vi "Write TDMS.vi"(8 "error in (no error)":errorcluster, 9 "Timed out? (False)":bool, 10 "Distance (m)":dbl, 11 "Parallax PING))) in":refnum<class "Parallax PING))).lvclass">) -> (0 "error out":errorcluster, 3 "Parallax PING))) out":refnum<class "Parallax PING))).lvclass">)   [LabVIEW 2013, in "Parallax PING))).lvclass"]
doc: "Writes data to the tdms file. Call Open TDMS VI before running this VI."
uses:
  Parallax PING))).lvclass
  Parallax PING))).lvclass/Parallax PING))).ctl
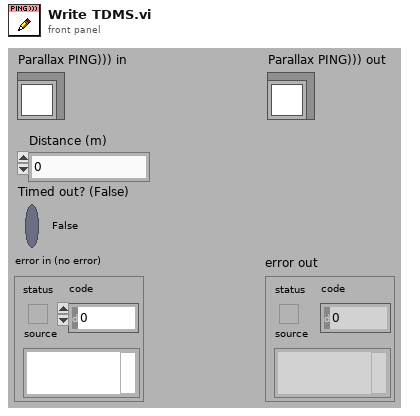
[diagram p1: front panel]
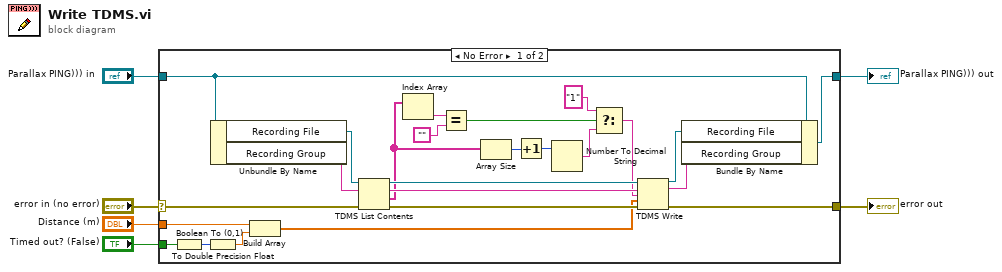
[diagram p0: block diagram]
diagram:
  n1 = case shown="No Error" "error in (no error)" {
    selector: "error in (no error)" -> [w24 w33]
    tunnel: [w31 w33] -> w2
    tunnel: [w27 w32] -> w3
    tunnel: "Parallax PING))) in" -> [w30 w32]
    tunnel: "Distance (m)" -> [w10 _]
    tunnel: "Timed out? (False)" -> [w9 _]
    frame No Error {
      n2 = Boolean To (0,1)(Boolean=w9) -> (0, 1=w8:i16)
      n3 = To Double Precision Float(number=w8) -> (double precision float=w7:dbl)
      n4 = Unbundle By Name(w30) -> ("Recording File"=w26:refnum<k34>, "Recording Group"=w25:string)
      n5 = Build Array(w10, w7) -> (w11:dbl[])
      n6 = TDMS List Contents(4:w24, 6:w25, 7:w26) -> (0:w19:errorcluster, 1:w14:string[], 2:w23:string, 3:w22:refnum<k34>)
      n7 = Index Array(array=w14) -> (element=w18:string)  [unwired: 1 in]
      n8 = Equal?(x=w18, y="") -> (x = y?=w16:bool)
      n9 = Array Size(array=w14) -> (size(s)=w21:i32)
      n10 = Increment(x=w21) -> (x+1=w20:i32)
      n11 = Number To Decimal String(number=w20) -> (decimal integer string=w13:string)  [unwired: 1 in]
      n12 = Select(t="1", s=w16, f=w13) -> (s? t:f=w12:string)
      n13 = TDMS Write(0:w22, 5:w23, 7:w12, 9:w11, 11:w19) -> (4:w29:refnum<k34>, 6:w28:string, 15:w31:errorcluster)  [unwired: 1 in, 1 out]
      n14 = Bundle By Name(cluster=w30, "Recording File"=w29, "Recording Group"=w28) -> (w27:refnum<class "Parallax PING))).lvclass">)
    }
    frame Error {
    }
  }
  "error out" <- w2
  "Parallax PING))) out" <- w3
